vi "Write Plugin.vi"(8 "error in (no error)":errorcluster, 9 "plugin values":T1={"type"="", "timing"={"priority"=0, "decimation"=0, "offset"=0}, "group ids"=[], "settings id"="", "thread count"=1}, 10 "id":string, 11 "Configuration Session in":refnum<class "Configuration Session.lvclass">) -> (0 "error out":errorcluster, 3 "Configuration Session out":refnum<class "Configuration Session.lvclass">, 4 "replaced?":bool)   [LabVIEW 2017, in "DSF Core.lvlib" / "Configuration Session.lvclass"]
doc: "Writes a value to a key in a specified section of the configuration data identified by <B>dsf refnum</B>. This VI modifies data in memory. To write data to disk, use the Close Config Data VI. Wire data to the <B>value</B> input to determine the polymorphic instance to use or manually select the instance."
uses:
  Configuration Session.lvclass
  Controls/DSF Plugin Info.ctl
  Controls/DSF Timing Info.ctl
  DSF Core.lvlib
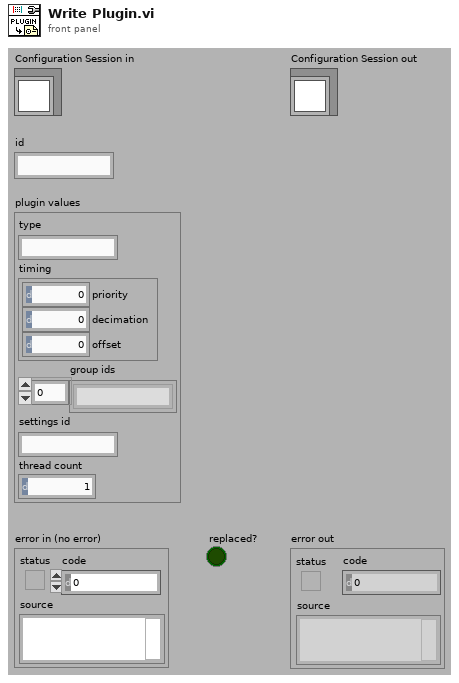
[diagram p1: front panel]
types:
  T1 = typedef "DSF Core.lvlib/DSF Plugin Info.ctl" = cluster{"type":string, "timing":T2, "group ids":string[], "settings id":string, "thread count":i32}
  T2 = typedef "DSF Core.lvlib/DSF Timing Info.ctl" = cluster{"priority":u64, "decimation":u64, "offset":u64}
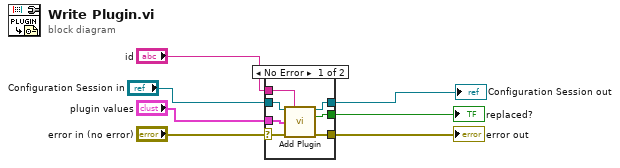
[diagram p0: block diagram]
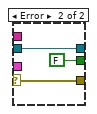
[diagram p2: hidden frame]
diagram:
  n1 = case shown="No Error" "error in (no error)" {
    selector: "error in (no error)" -> [w11 w17]
    tunnel: [w12 w17] -> w6
    tunnel: "id" -> [w14 _]
    tunnel: [w13 FALSE ("key exists?")] -> w4
    tunnel: "Configuration Session in" -> [w10 w15]
    tunnel: [w9 w15] -> w1
    tunnel: "plugin values" -> [w8 _]
    frame No Error {
      n2 = call "Add Plugin.vi"("Configuration Session in"=w10, "id"=w14, "values"=w8, "error in (no error)"=w11) -> ("Configuration Session out"=w9:refnum<class "Configuration Session.lvclass">, "exists?"=w13:bool, "error out"=w12:errorcluster)  [unwired: 2 in, 7 out]
    }
    frame Error {
    }
  }
  "error out" <- w6
  "replaced?" <- w4
  "Configuration Session out" <- w1
